vi "Read Angle To Turn.vi"(8 "error in (no error)":errorcluster, 11 "TurnInstruction in":refnum<class "TurnInstruction.lvclass">) -> (0 "error out":errorcluster, 2 "Angle To Turn":dbl, 3 "TurnInstruction out":refnum<class "TurnInstruction.lvclass">)   [LabVIEW 2015, in "TurnInstruction.lvclass"]
uses:
  TurnInstruction.lvclass
  TurnInstruction.lvclass/TurnInstruction.ctl
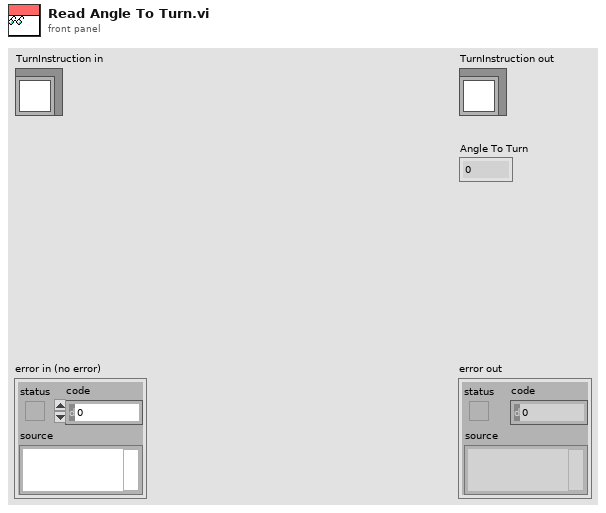
[diagram p1: front panel]
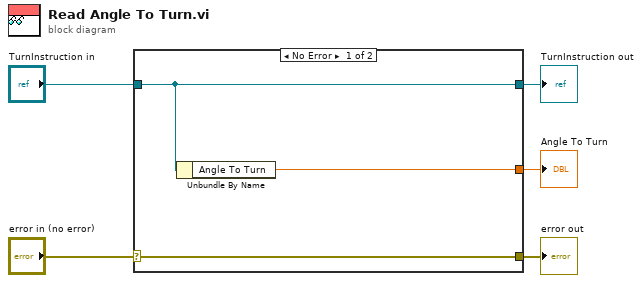
[diagram p0: block diagram]
diagram:
  n1 = case shown="No Error" "error in (no error)" {
    selector: "error in (no error)" -> [w8 w9]
    tunnel: [w8 w9] -> w4
    tunnel: [w7 w10] -> w2
    tunnel: "TurnInstruction in" -> [w7 w10]
    tunnel: [w6 _] -> w1
    frame No Error {
      n2 = Unbundle By Name(w7) -> ("Angle To Turn"=w6:dbl)
    }
    frame Error {
    }
  }
  "error out" <- w4
  "TurnInstruction out" <- w2
  "Angle To Turn" <- w1
